vi "Add Item To Listbox.vi"(0 "Display State In":T1, 5 "Item Name":string, 9 "Container State":T2, 11 "error in (no error)":errorcluster) -> (4 "Display State Out":T1, 15 "error out":errorcluster)   [LabVIEW 2011, in "X Listbox-Solution.xctl"]
doc: "This is a method for the X Listbox. Details about implementation can be found in the course manual.\n\nAAL 9/09"
uses:
  X Listbox-Solution.xctl
  <vilib>/_xctls/Container State.ctl
  Abilities/X Listbox State.ctl
  <vilib>/_xctls/XControlSupport.lvlib
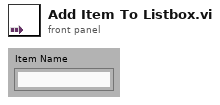
[diagram p1: front panel]
types:
  T1 = typedef "X Listbox-Solution.xctl/X Listbox State.ctl" = cluster{"# Items":i32, "Names":string[]}
  T2 = typedef "XControlSupport.lvlib/Container State.ctl" = cluster{"Indicator?":bool, "Run Mode?":bool, " Refnum":refnum<vi>}
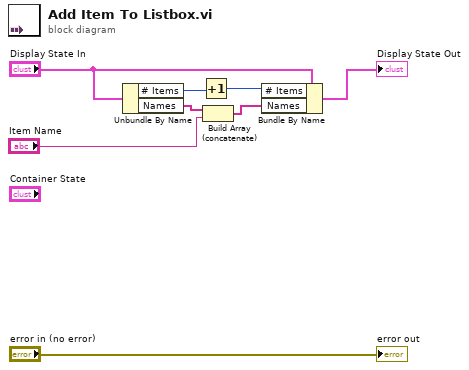
[diagram p0: block diagram]
diagram:
  n1 = Unbundle By Name("Display State In") -> ("# Items"=w5:i32, "Names"=w3:string[])
  n2 = Increment(x=w5) -> (x+1=w4:i32)
  n3 = Build Array (concatenate)(w3, "Item Name") -> (w1:string[])
  n4 = Bundle By Name(cluster="Display State In", "# Items"=w4, "Names"=w1) -> (→"Display State Out":T1)
  "error out" <- "error in (no error)"
